vi "Configure Messages.vi"(8 "error in (no error)":errorcluster, 10 "Messages":string[](array[string]), 11 "Debugger In":refnum<class "Debugger.lvclass">) -> (0 "error out":errorcluster, 3 "Debugger Out":refnum<class "Debugger.lvclass">)   [LabVIEW 2020, in "Debugger.lvclass"]
uses:
  Debugger.lvclass
  C:/Users/anton/Documents/GitHub/triarc-debugger/source/Process/Debug Process.lvclass
  Process/Debug Process.lvclass/Debug Process.ctl
  <vilib>/Utility/error.llb/Clear Errors.vi
  Filter by Message/Filter by Message.lvclass
  C:/Users/anton/Documents/GitHub/triarc-debugger/source/Filter/Filter.lvclass
  <vilib>/Utility/error.llb/Error Cluster From Error Code.vi
  Debugger.lvclass/Debugger.ctl
  Process/Debug Process.lvclass
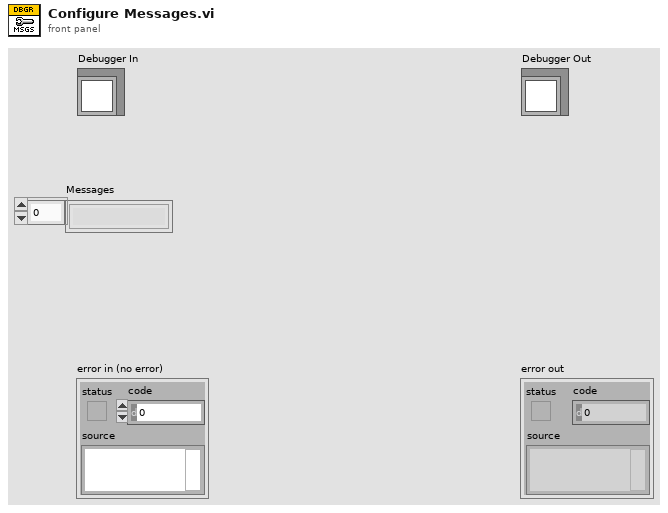
[diagram p1: front panel]
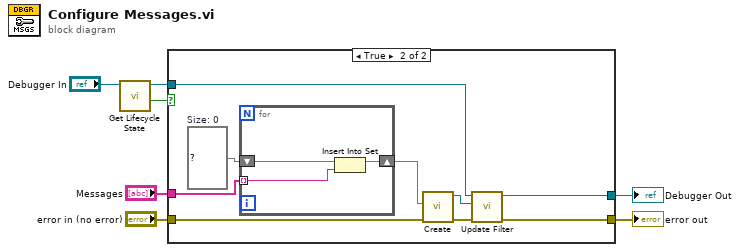
[diagram p0: block diagram]
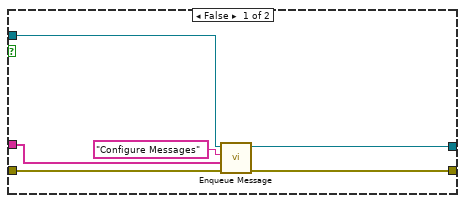
[diagram p2: hidden frame]
diagram:
  n1 = call "Get Lifecycle State.vi"("Process In"="Debugger In") -> ("In Process Loop?"=w1:bool, "Process Out"=w2:refnum<class "Debugger.lvclass">)  [unwired: 7 in, 2 out]
  n2 = case shown="True" w1 {
    tunnel: "error in (no error)" -> [w13 w21]
    tunnel: [w12 w20] -> w6
    tunnel: [w11 w15] -> w4
    tunnel: "Messages" -> [w9 w22]
    tunnel: w2 -> [w8 w14]
    frame False {
      n3 = call "Enqueue Message.vi"("error in (no error)"=w13, "Message Data"=w9, "Message"="Configure Messages", "Process In"=w8) -> ("error out"=w12:errorcluster, "Process Out"=w11:refnum<class "Debugger.lvclass">)  [unwired: 6 in]
    }
    frame True {
      w18 = set{string} {}  # Size: 0
      n4 = for {
        shift-right: [w24] -> w19
        shift-left: w18 -> [w25]
        tunnel: w22 -> [w23] mode=indexing
        n5 = Insert Into Set(10:w23, 11:w25) -> (3:w24:set{string})  [unwired: 1 out]
      }
      n6 = call "Create.vi"("error in (no error)"=w21, "Messages"=w19) -> ("error out"=w16:errorcluster, "Filter by Process out"=w17:refnum<class "Filter by Message.lvclass">)  [unwired: 8 in]
      n7 = call "Update Filter.vi"("error in (no error)"=w16, "Filter in"=w17, "Debugger in"=w14) -> ("error out"=w20:errorcluster, "Debugger out"=w15:refnum<class "Debugger.lvclass">)  [unwired: 7 in]
    }
  }
  "error out" <- w6
  "Debugger Out" <- w4
